vi "DebugMove.vi"() -> ()   [LabVIEW 2017]
uses:
  Global Encoder.vi
panel:
  out "Count Encode 2":dbl
  out "Count Encode 1":dbl
  in  "Start":bool
  in  "stop":bool
  in  "Encode":dbl
  in  "Speed":dbl
  in  "Delay":dbl
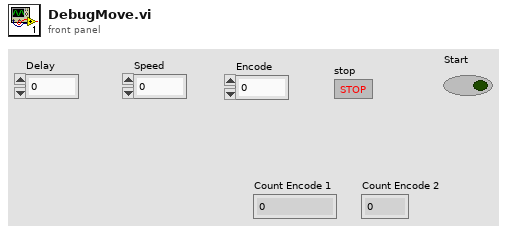
[diagram p1: front panel]
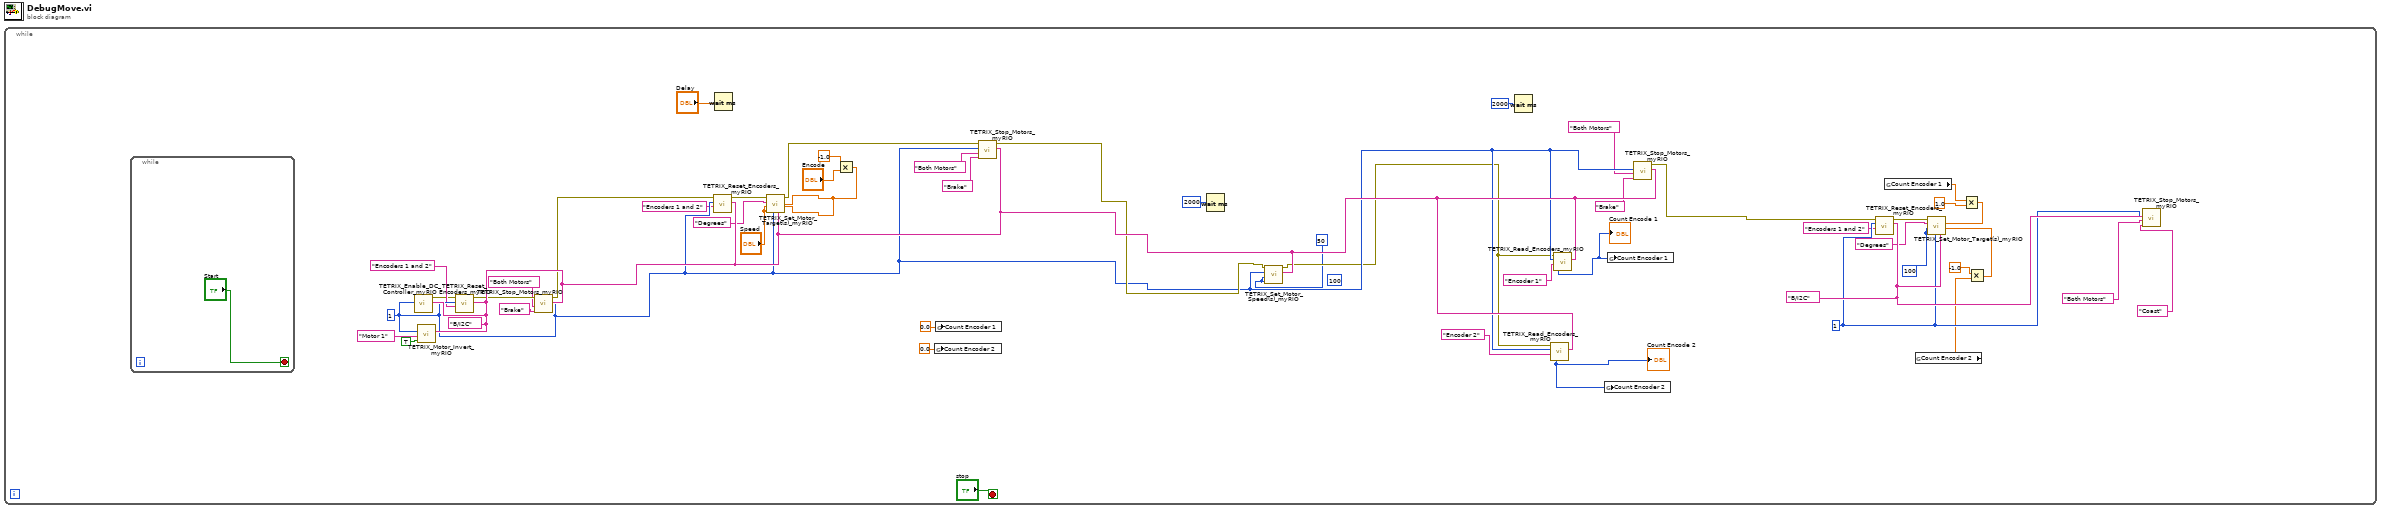
[diagram p0: block diagram]
diagram:
  n1 = while {
    stop <- "stop" stop-if-true
    w1 = i16 100 ("Motor 1 Contant Speed (Degrees per Second)")
    w11 = u8 1 ("Controller ID#  (I2C Address)")
    w14 = tag "B/I2C" ("myRIO MXP Port A/B")
    w22 = 50 ("Motor 1 Encoder Target")
    (unwired) i16 100 ("Motor 1 Contant Speed (Degrees per Second)")
    w48 = tag "B/I2C" ("myRIO MXP Port A/B")
    w44 = u8 1 ("Controller ID#  (I2C Address)")
    n2 = while {
      stop <- "Start" stop-if-true
    }
    n3 = call <vilib>:"TETRIX_Enable_DC_Controller_myRIO.vi"("myRIO MXP Port A/B"=w48, "Controller ID#  (I2C Address)"=w44) -> ("Error/Flow Out"=w38:errorcluster)  [unwired: 5 in]
    n4 = call <vilib>:"TETRIX_Motor_Invert_myRIO.vi"("myRIO MXP Port A/B"=w48, "Invert State"=TRUE, "Select Channel"="Motor 1", "Controller ID#  (I2C Address)"=w44) -> ()  [unwired: 3 in, 1 out]
    n5 = call <vilib>:"TETRIX_Reset_Encoders_myRIO.vi"("myRIO MXP Port A/B"=w48, "Select Encoder"="Encoders 1 and 2", "Controller ID#  (I2C Address)"=w44, "Error/Flow In"=w38) -> ("Error/Flow Out"=w37:errorcluster)  [unwired: 3 in]
    n6 = call <vilib>:"TETRIX_Stop_Motors_myRIO.vi"("myRIO MXP Port A/B"=w48, "Stop Mode"="Brake", "Select Channel"="Both Motors", "Controller ID#  (I2C Address)"=w44, "Error/Flow In"=w37) -> ("Error/Flow Out"=w46:errorcluster)  [unwired: 2 in]
    n7 = call <vilib>:"TETRIX_Reset_Encoders_myRIO.vi"("myRIO MXP Port A/B"=w48, "Select Encoder"="Encoders 1 and 2", "Controller ID#  (I2C Address)"=w44, "Error/Flow In"=w46) -> ("Error/Flow Out"=w35:errorcluster)  [unwired: 3 in]
    n8 = Wait (ms)(milliseconds to wait="Delay") -> ()  [unwired: 1 out]
    n9 = Multiply(x=-1.0, y="Encode") -> (x*y=w28:dbl)
    n10 = call <vilib>:"TETRIX_Set_Motor_Target(s)_myRIO.vi"("Motor 2 Encoder Target"=w28, "Motor 1 Encoder Target"=w28, "myRIO MXP Port A/B"=w48, "Controller ID#  (I2C Address)"=w44, "Motor 2 Constant Speed (Degrees per Second)"="Speed", "Motor 1 Contant Speed (Degrees per Second)"="Speed", "Encoder Units"="Degrees", "Error/Flow In"=w35) -> ("Error/Flow Out"=w45:errorcluster)  [unwired: 1 in]
    n11 = global write "Global Encoder.vi" "Count Encoder 2"(0.0 ("Count Encoder 1")) -> ()
    n12 = global write "Global Encoder.vi" "Count Encoder 1"(0.0 ("Count Encoder 1")) -> ()
    n13 = call <vilib>:"TETRIX_Stop_Motors_myRIO.vi"("myRIO MXP Port A/B"=w48, "Stop Mode"="Brake", "Select Channel"="Both Motors", "Controller ID#  (I2C Address)"=w44, "Error/Flow In"=w45) -> ("Error/Flow Out"=w47:errorcluster)  [unwired: 2 in]
    n14 = Wait (ms)(milliseconds to wait=u32 2000 ("millisecond timer value")) -> ()  [unwired: 1 out]
    n15 = call <vilib>:"TETRIX_Set_Motor_Speed(s)_myRIO.vi"("myRIO MXP Port A/B"=w48, "Motor 2 Speed (Degrees per second). Sign (+/-)  sets direction."=w22, "Motor 1 Speed (Degrees per second). Sign (+/-)  sets direction."=w22, "Controller ID#  (I2C Address)"=w44, "Error/Flow In"=w47) -> ("Error/Flow Out"=w43:errorcluster)  [unwired: 2 in]
    n16 = Wait (ms)(milliseconds to wait=u32 2000 ("millisecond timer value")) -> ()  [unwired: 1 out]
    n17 = call <vilib>:"TETRIX_Read_Encoders_myRIO.vi"("myRIO MXP Port A/B"=w48, "Select Encoder"="Encoder 2", "Controller ID#  (I2C Address)"=w44, "Error/Flow In"=w43) -> ("Encoder Output"=w18:i32)  [unwired: 2 in, 1 out]
    "Count Encode 2" <- w18
    n18 = call <vilib>:"TETRIX_Read_Encoders_myRIO.vi"("myRIO MXP Port A/B"=w48, "Select Encoder"="Encoder 1", "Controller ID#  (I2C Address)"=w44, "Error/Flow In"=w43) -> ("Encoder Output"=w16:i32)  [unwired: 2 in, 1 out]
    "Count Encode 1" <- w16
    n19 = global write "Global Encoder.vi" "Count Encoder 2"(w18) -> ()
    n20 = global write "Global Encoder.vi" "Count Encoder 1"(w16) -> ()
    n21 = call <vilib>:"TETRIX_Stop_Motors_myRIO.vi"("myRIO MXP Port A/B"=w48, "Stop Mode"="Brake", "Select Channel"="Both Motors", "Controller ID#  (I2C Address)"=w44) -> ("Error/Flow Out"=w49:errorcluster)  [unwired: 3 in]
    n22 = call <vilib>:"TETRIX_Reset_Encoders_myRIO.vi"("myRIO MXP Port A/B"=w14, "Select Encoder"="Encoders 1 and 2", "Controller ID#  (I2C Address)"=w11, "Error/Flow In"=w49) -> ("Error/Flow Out"=w10:errorcluster)  [unwired: 3 in]
    n23 = global read "Global Encoder.vi" "Count Encoder 1"() -> (w7:dbl)
    n24 = global read "Global Encoder.vi" "Count Encoder 2"() -> (w5:dbl)
    n25 = Multiply(x=w7, y=1.0) -> (x*y=w6:dbl)
    n26 = Multiply(x=-1.0 ("y"), y=w5) -> (x*y=w2:dbl)
    n27 = call <vilib>:"TETRIX_Set_Motor_Target(s)_myRIO.vi"("Motor 2 Encoder Target"=w2, "Motor 1 Encoder Target"=w6, "myRIO MXP Port A/B"=w14, "Controller ID#  (I2C Address)"=w11, "Motor 2 Constant Speed (Degrees per Second)"=w1, "Motor 1 Contant Speed (Degrees per Second)"=w1, "Encoder Units"="Degrees", "Error/Flow In"=w10) -> ()  [unwired: 1 in, 1 out]
    n28 = call <vilib>:"TETRIX_Stop_Motors_myRIO.vi"("myRIO MXP Port A/B"=w14, "Stop Mode"="Coast", "Select Channel"="Both Motors", "Controller ID#  (I2C Address)"=w11) -> ()  [unwired: 3 in, 1 out]
  }
